vi "UTILITY Elapsed Time General Info.vi"(5 "Add Elapsed Time (hrs)":bool, 6 "precision (6)":i16=6, 7 "Add Software Elapsed Time":bool, 8 "Error In":errorcluster, 10 "Software Elapsed Time":dbl format="%<%H:%M:%S>t", 11 "Elapsed Time (sec)":dbl) -> (0 "Error Out":errorcluster, 1 "Main Loop Rate":dbl format="%0.2f", 2 "Total Array":string[][](array[string]), 3 "Elapsed Time":dbl, 4 "Main Start":dbl format="%.2f")   [LabVIEW 2018]
uses:
  <vilib>/ptbypt/NI_PtbyPt.lvlib
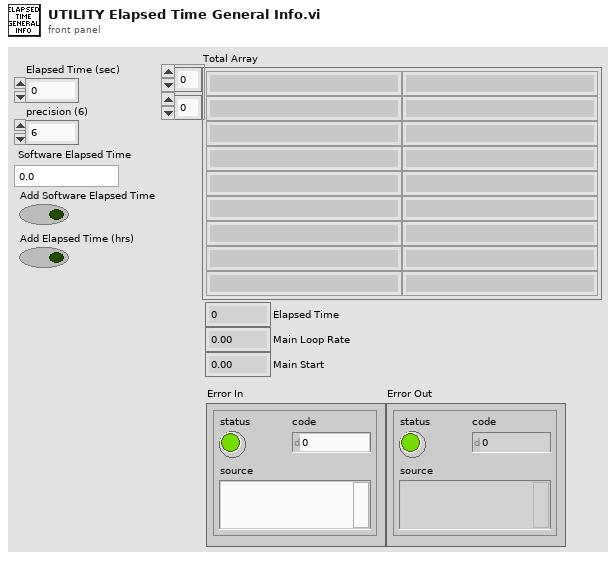
[diagram p1: front panel]
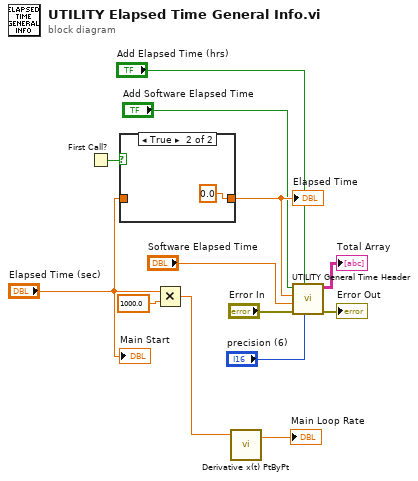
[diagram p0: block diagram]
diagram:
  n1 = First Call?() -> (First Call?: T/F=w13:bool)
  n2 = case shown="True" w13 {
    tunnel: [w14 0.0 ("Start")] -> w11
    tunnel: "Elapsed Time (sec)" -> [w14 _]
    frame False {
    }
    frame True {
    }
  }
  "Elapsed Time" <- w11
  n3 = Multiply(x="Elapsed Time (sec)", y=1000.0) -> (x*y=w9:dbl)
  n4 = call <vilib>:"Derivative x(t) PtByPt.vi"("x"=w9) -> ("dx/dt"=→"Main Loop Rate":dbl)  [unwired: 3 in, 1 out]
  n5 = call "UTILITY General Time Header.vi"("precision (6)"="precision (6)", "Add Elapsed Time (hrs)"="Add Elapsed Time (hrs)", "Error In"="Error In", "Software Elapsed Time"="Software Elapsed Time", "Elapsed Time"=w11, "Add Software Elapsed Time"="Add Software Elapsed Time") -> ("Error Out"=→"Error Out":errorcluster, "Total Array"=→"Total Array":string[][])  [unwired: 4 in]
  "Main Start" <- "Elapsed Time (sec)"
